vi "Save Local Images.vi"(2 "Save Images":bool, 3 "Image Pathnames":path[](array[path]), 4 "Camera Names":string[](array[string])) -> (0 "error out":errorcluster, 1 "Filenames out":path[](array[path]))   [LabVIEW 2022 SP3]
uses:
  Anemometry Sub Vis/Globals/Preference_global.vi
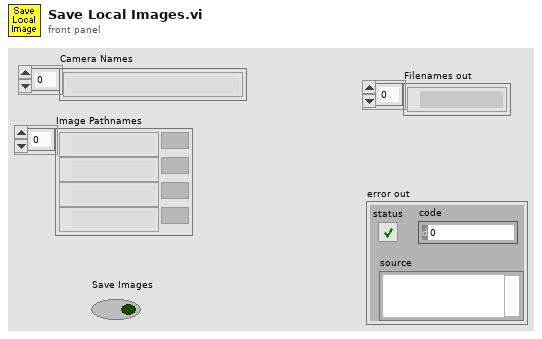
[diagram p1: front panel]
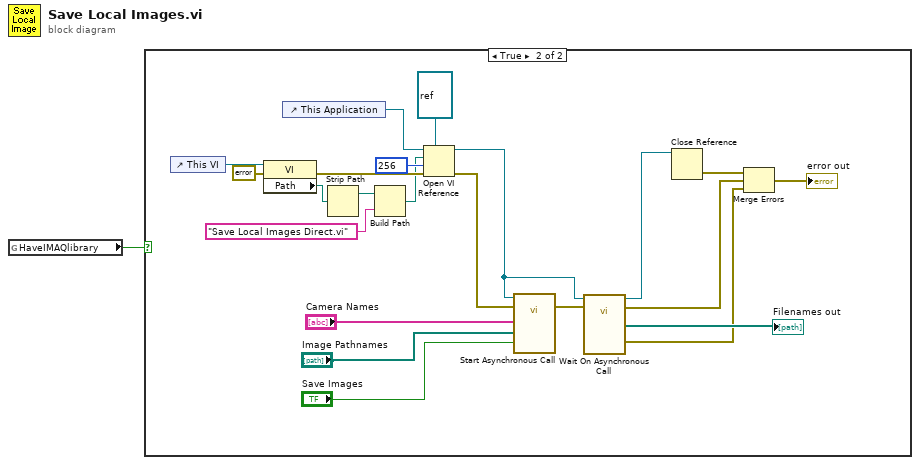
[diagram p0: block diagram]
diagram:
  n1 = global read "Preference_global.vi" "HaveIMAQlibrary"() -> (w1:bool)
  n2 = case shown="True" w1 {
    frame False {
    }
    frame True {
      n3 = control-ref of="This VI"() -> (w13:refnum<vi>)
      n4 = property class="VI"(reference=w13, error in=errorcluster {"status"=FALSE, "code"=0, "source"=""} ("error in (no error)")) -> (error out=w16:errorcluster, "Path"=w20:path)  [unwired: 1 out]
      n5 = control-ref of="This Application"() -> (w18:refnum<vi>)
      n6 = Strip Path(path=w20) -> (stripped path=w21:path)  [unwired: 1 out]
      n7 = Build Path(base path=w21, name or relative path="Save Local Images Direct.vi") -> (appended path=w15:path)
      n8 = Open VI Reference(type specifier VI Refnum (for type only)=refnum<vi> refnum, application reference (local)=w18, vi path=w15, options=256, error in (no error)=w16) -> (vi reference=w2:refnum<vi>, error out=w22:errorcluster)  [unwired: 1 in]
      n9 = call-by-ref "Start Asynchronous Call"(reference=w2, error in=w22, "Save Images"="Save Images", "Image Pathnames"="Image Pathnames", "Camera Names"="Camera Names") -> (error out=w3:errorcluster)  [unwired: 3 out]
      n10 = call-by-ref "Wait On Asynchronous Call"(reference=w2, error in=w3) -> (reference out=w23:refnum<vi>, error out=w5:errorcluster, 0:"error out"=w4:errorcluster, "Filenames out"=→"Filenames out":path[])  [unwired: 3 in]
      n11 = Close Reference(reference=w23) -> (error out=w11:errorcluster)  [unwired: 1 in]
      n12 = Merge Errors(w11, w5, w4) -> (→"error out":errorcluster)
    }
  }
